vi "Loop Frequency.vi"() -> (0 "Loop Rate (Hz)":u32)   [LabVIEW 2020, in "Device.lvlib"]
doc: "Place this VI in a loop to calculate the loop rate. Using multiple copies of this VI in an application is not supported and will return incorrect results."
uses:
  Device.lvlib
  <vilib>/ptbypt/NI_PtbyPt.lvlib
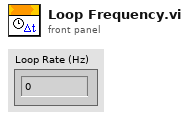
[diagram p1: front panel]
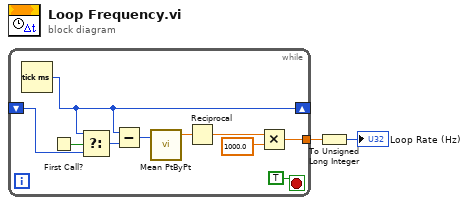
[diagram p0: block diagram]
diagram:
  n1 = while {
    shift-right: [w3] -> _
    shift-left: _ -> [w7]
    tunnel: [w4] -> w2
    stop <- TRUE stop-if-true
    n2 = Tick Count (ms)() -> (millisecond timer value=w3:u32)
    n3 = First Call?() -> (First Call?: T/F=w12:bool)
    n4 = Select(t=w3, s=w12, f=w7) -> (s? t:f=w11:u32)
    n5 = Subtract(x=w3, y=w11) -> (x-y=w10:u32)
    n6 = call <vilib>:"Mean PtByPt.vi"("x"=w10) -> ("mean"=w9:dbl)  [unwired: 3 in, 1 out]
    n7 = Reciprocal(x=w9) -> (1/x=w5:dbl)
    n8 = Multiply(x=w5, y=1000.0) -> (x*y=w4:dbl)
  }
  n9 = To Unsigned Long Integer(number=w2) -> (unsigned 32bit integer=→"Loop Rate (Hz)":u32)
